vi "Финал.vi"() -> ()   [LabVIEW 2017]
panel:
  out "Result":T1
  in  "-":bool
  in  "R":bool
  in  "C":bool
  in  "Ввод":T2
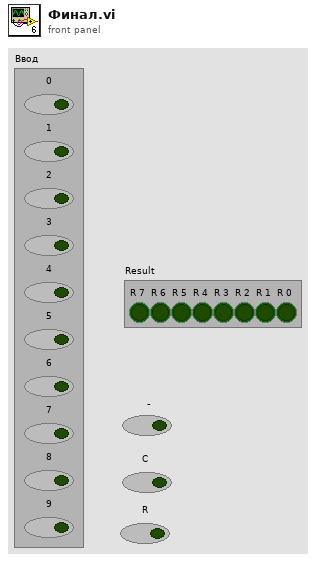
[diagram p1: front panel]
types:
  T1 = cluster{"R 7":bool, "R 6":bool, "R 5":bool, "R 4":bool, "R 3":bool, "R 2":bool, "R 1":bool, "R 0":bool}
  T2 = cluster{"0":bool, "1":bool, "2":bool, "3":bool, "4":bool, "5":bool, "6":bool, "7":bool, "8":bool, "9":bool}
  T3 = cluster{"Boolean 7":bool, "Boolean 8":bool, "Boolean 9":bool, "Boolean 10":bool}
  T4 = cluster{"Boolean 2":bool, "Boolean 3":bool, "Boolean 4":bool, "Boolean 5":bool}
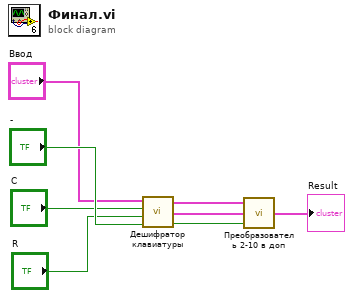
[diagram p0: block diagram]
diagram:
  n1 = call "Дешифратор клавиатуры.vi"("-"="-", "R"="R", "C"="C", "Input"="Ввод") -> ("-"=w4:bool, "Един"=w3:T3, "Дес"=w2:T4)
  n2 = call "Преобразователь 2-10 в доп.vi"("-"=w4, "H"=w3, "L"=w2) -> ("R"=→"Result":T1)
